vi "main.vi"() -> ()   [LabVIEW 2018]
uses:
  ControlEstados3.ctl
  <vilib>/MakerHub/LINX/Public/Peripherals/PWM/PWM Set Duty Cycle 1 Chan.vi
  <vilib>/MakerHub/LINX/Public/Utilities/Open Serial.vi
  <vilib>/MakerHub/LINX/Public/Peripherals/PWM/PWM Set Duty Cycle N Chans.vi
  <vilib>/MakerHub/LINX/LMH-LINX.lvlib
panel:
  out "Estado":T1
  in  "Máquina de estado":enum32{"LM35 RGB", "Hall sensor"}(tab)
  in  "Temperatura optima (led azul)":dbl=0.25 format="%#_13g"
  in  "Temperatura limite":dbl
  out "Color Box 2":u32(colorbox)
  out "Thermometer":dbl(slide) scale=0.0..100.0
  in  "lm35":bool
  in  "Parar lm35":bool
  out "hall indicator":bool
  in  "hall":bool
  in  "Parar hall":bool
  in  "Serial Port":refnum<visa-resource-name>="N/A"
  in  "stop":bool
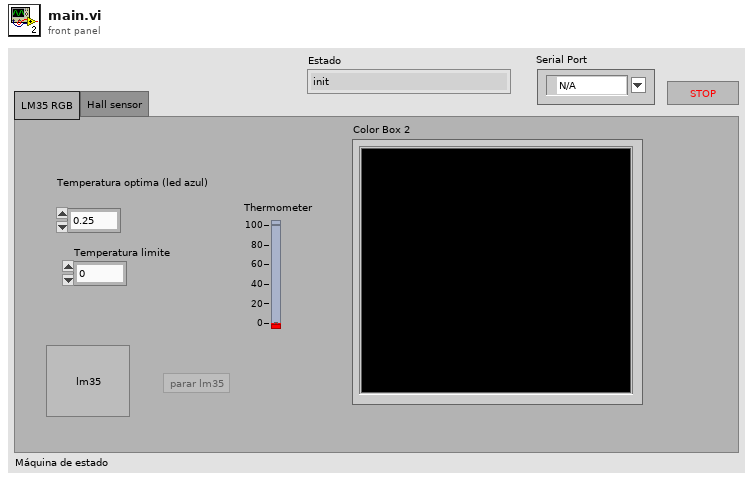
[diagram p1: front panel]
types:
  T1 = typedef "ControlEstados3.ctl" = enum16{"init", "wait for user event", "stop", "lm35", "hall"}
  T2 = enum8{"Enabled", "Disabled", "Disabled and Grayed Out"}
  T3 = typedef "LMH-LINX.lvlib/LINX Ref.ctl" = cluster{"IO":T4, "Interface":T5, "LINX Device Config":T6}
  T4 = typedef "LMH-LINX.lvlib/Platform.ctl" = enum16{"Remote", "Local"}
  T5 = typedef "LMH-LINX.lvlib/Interface.ctl" = enum16{"Serial", "TCP"}
  T6 = typedef "LMH-LINX.lvlib/Device.lvlib/LINX Device Config.ctl" = cluster{"Interface":T5, "COM Port":refnum<visa-resource-name>, "TCP Configuration":T7, "Device Family":u8, "Device ID":u8, "Device Name":string, "TCP Ref":refnum<k5>, "Channels":T8}
  T7 = typedef "LMH-LINX.lvlib/Device.lvlib/TCP Config.ctl" = cluster{"IP Address":string, "Port":u16}
  T8 = typedef "LMH-LINX.lvlib/Channels.ctl" = cluster{"DI":u8[], "DO":u8[], "AI":u8[], "AO":u8[], "PWM":u8[], "QE":u8[], "UART":u8[], "I2C 2":u8[], "SPI":u8[], "CAN":u8[], "Servo":u8[], "AI Ref (V)":dbl, "AI Resolution (Bits)":u8, "AO Ref (V)":dbl, "AO Resolution (Bits)":u8}
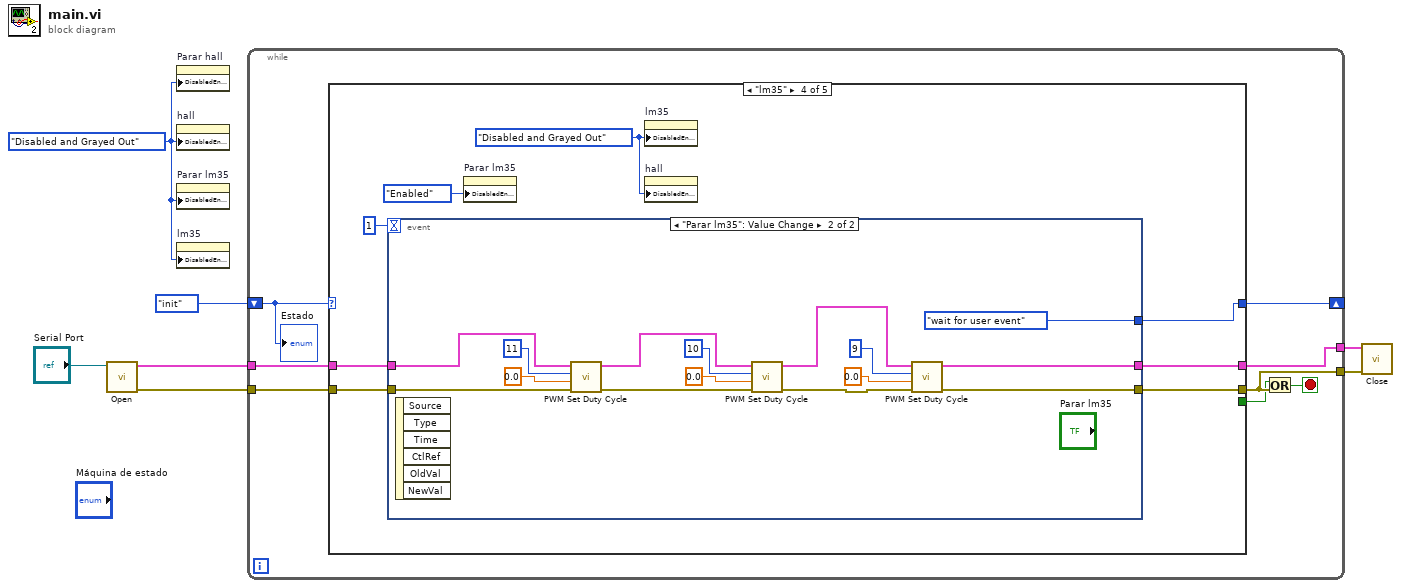
[diagram p0: block diagram]
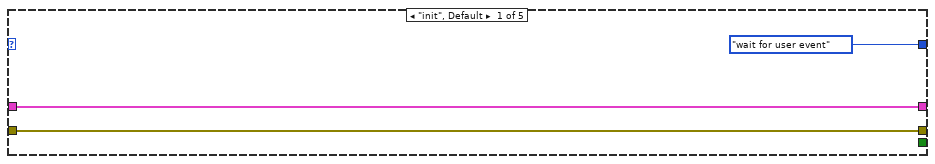
[diagram p2: hidden frame]
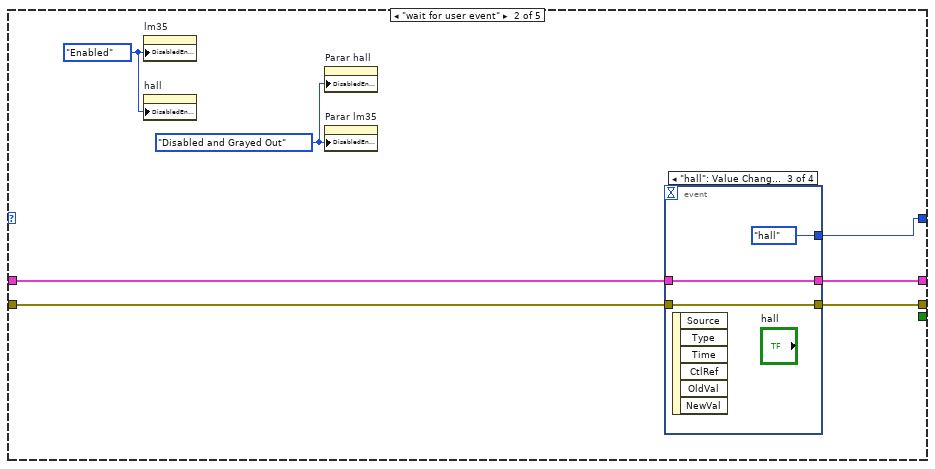
[diagram p3: hidden frame]
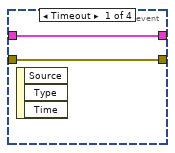
[diagram p4: hidden frame]
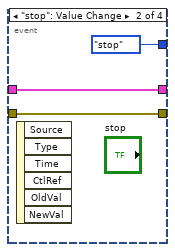
[diagram p5: hidden frame]
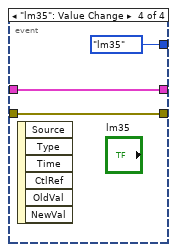
[diagram p6: hidden frame]
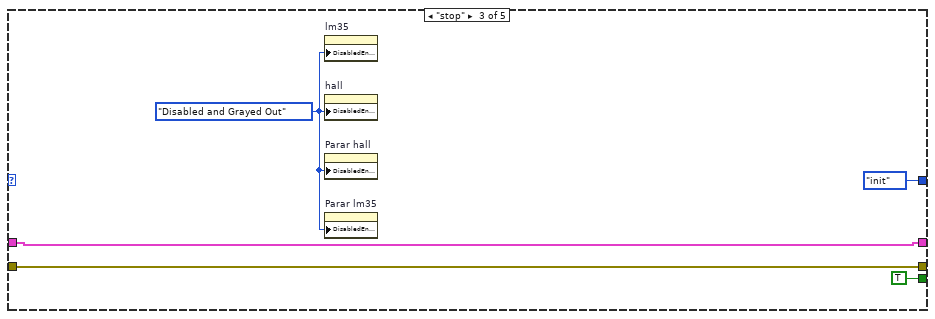
[diagram p7: hidden frame]
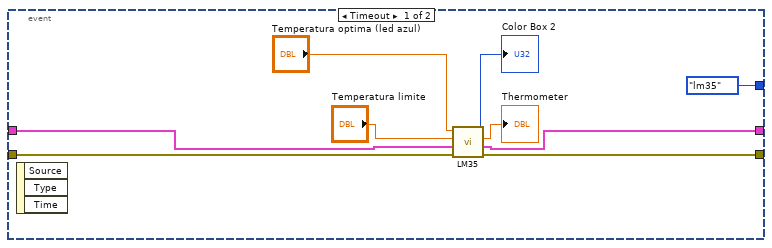
[diagram p8: hidden frame]
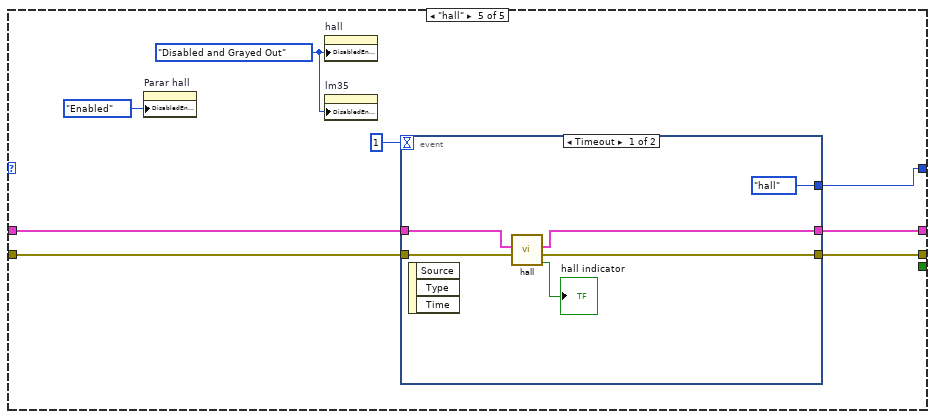
[diagram p9: hidden frame]
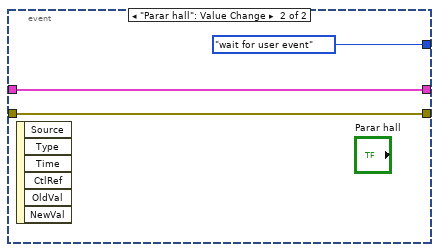
[diagram p10: hidden frame]
diagram:
  w1 = T2."Disabled and Grayed Out" ("Disabled")
  n1 = call-poly <vilib>:"Open.vi"("Serial Port"="Serial Port") -> ("Error Out"=w4:errorcluster, "LINX Resource"=w5:T3)  [unwired: 8 in, 1 out]
  n2 = property on="Parar hall" class="Bool"("DisabledEnum"=w1) -> ()  [unwired: 2 in, 2 out]
  n3 = property on="hall" class="Bool"("DisabledEnum"=w1) -> ()  [unwired: 2 in, 2 out]
  n4 = property on="Parar lm35" class="Bool"("DisabledEnum"=w1) -> ()  [unwired: 2 in, 2 out]
  n5 = property on="lm35" class="Bool"("DisabledEnum"=w1) -> ()  [unwired: 2 in, 2 out]
  n6 = while {
    shift-right: [w15] -> _
    shift-left: ControlEstados3."init" -> [w11]
    tunnel: w5 -> [w14]
    tunnel: w4 -> [w13]
    tunnel: [w12] -> w3
    tunnel: [w10] -> w2
    stop <- w8 stop-if-true
    n7 = case shown="\"lm35\"" w11 {
      tunnel: [ControlEstados3."wait for user event" w25 ControlEstados3."init" w49 w81] -> w15
      tunnel: [_ _ TRUE _ _] -> w9
      tunnel: w14 -> [w17 w23 w39 w46 w79]
      tunnel: w13 -> [w16 w21 w38 w44 w78]
      tunnel: [w17 w24 w39 w47 w77] -> w12
      tunnel: [w16 w22 w38 w45 w76] -> w10
      frame "init", Default {
      }
      frame "wait for user event" {
        w19 = T2."Disabled and Grayed Out" ("Disabled")
        w20 = T2."Enabled" ("Disabled")
        n8 = property on="lm35" class="Bool"("DisabledEnum"=w20) -> ()  [unwired: 2 in, 2 out]
        n9 = property on="hall" class="Bool"("DisabledEnum"=w20) -> ()  [unwired: 2 in, 2 out]
        n10 = property on="Parar hall" class="Bool"("DisabledEnum"=w19) -> ()  [unwired: 2 in, 2 out]
        n11 = property on="Parar lm35" class="Bool"("DisabledEnum"=w19) -> ()  [unwired: 2 in, 2 out]
        n12 = event shown="[2] \"hall\": Value Change" {
          selector: _ -> [_ _ _ _]
          dyn-events: _ -> [_ _ _ _]
          timeout: _ -> [_ _ _ _]
          tunnel: [_ ControlEstados3."stop" ControlEstados3."hall" ControlEstados3."lm35"] -> w25
          tunnel: [w27 w29 w32 w35] -> w24
          tunnel: w23 -> [w27 w29 w32 w35]
          tunnel: [w26 w28 w31 w34] -> w22
          tunnel: w21 -> [w26 w28 w31 w34]
          event Timeout {
            n13 = event-data() -> ()  [unwired: 1 in, 3 out]
          }
          event "stop": Value Change {
            n14 = event-data() -> ()  [unwired: 1 in, 6 out]
          }
          event "hall": Value Change {
            n15 = event-data() -> ()  [unwired: 1 in, 6 out]
          }
          event "lm35": Value Change {
            n16 = event-data() -> ()  [unwired: 1 in, 6 out]
          }
        }
      }
      frame "stop" {
        w37 = T2."Disabled and Grayed Out" ("Disabled")
        n17 = property on="lm35" class="Bool"("DisabledEnum"=w37) -> ()  [unwired: 2 in, 2 out]
        n18 = property on="hall" class="Bool"("DisabledEnum"=w37) -> ()  [unwired: 2 in, 2 out]
        n19 = property on="Parar hall" class="Bool"("DisabledEnum"=w37) -> ()  [unwired: 2 in, 2 out]
        n20 = property on="Parar lm35" class="Bool"("DisabledEnum"=w37) -> ()  [unwired: 2 in, 2 out]
      }
      frame "lm35" {
        w42 = T2."Disabled and Grayed Out" ("Disabled")
        n21 = event shown="[1] \"Parar lm35\": Value Change" {
          selector: _ -> [_ _]
          dyn-events: _ -> [_ _]
          timeout: 1 -> [_ _]
          tunnel: [ControlEstados3."lm35" ControlEstados3."wait for user event"] -> w49
          tunnel: [w51 w63] -> w47
          tunnel: w46 -> [w55 w66]
          tunnel: [w50 w59] -> w45
          tunnel: w44 -> [w54 w62]
          event Timeout {
            n22 = event-data() -> ()  [unwired: 1 in, 3 out]
            n23 = call "LM35.vi"("Error In"=w54, "LINX Resource"=w55, "temperatura limite"="Temperatura limite", "Temperatura optima (led azul)"="Temperatura optima (led azul)") -> ("Error Out"=w50:errorcluster, "LINX Resource 2"=w51:T3, "Thermometer"=→"Thermometer":dbl, "Color Box 2"=→"Color Box 2":u32)  [unwired: 4 in]
          }
          event "Parar lm35": Value Change {
            n24 = event-data() -> ()  [unwired: 1 in, 6 out]
            n25 = call-poly <vilib>:"PWM Set Duty Cycle.vi"("Error In"=w62, "Duty Cycle (0-1)"=0.0, "PWM Channel"=u8 11, "LINX Resource"=w66) -> ("Error Out"=w61:errorcluster, "LINX Resource"=w65:T3)  [unwired: 6 in]
            n26 = call-poly <vilib>:"PWM Set Duty Cycle.vi"("Error In"=w61, "Duty Cycle (0-1)"=0.0, "PWM Channel"=u8 10, "LINX Resource"=w65) -> ("Error Out"=w60:errorcluster, "LINX Resource"=w64:T3)  [unwired: 6 in]
            n27 = call-poly <vilib>:"PWM Set Duty Cycle.vi"("Error In"=w60, "Duty Cycle (0-1)"=0.0, "PWM Channel"=u8 9, "LINX Resource"=w64) -> ("Error Out"=w59:errorcluster, "LINX Resource"=w63:T3)  [unwired: 6 in]
          }
        }
        n28 = property on="Parar lm35" class="Bool"("DisabledEnum"=T2."Enabled" ("Disabled")) -> ()  [unwired: 2 in, 2 out]
        n29 = property on="lm35" class="Bool"("DisabledEnum"=w42) -> ()  [unwired: 2 in, 2 out]
        n30 = property on="hall" class="Bool"("DisabledEnum"=w42) -> ()  [unwired: 2 in, 2 out]
      }
      frame "hall" {
        w74 = T2."Disabled and Grayed Out" ("Disabled")
        n31 = property on="Parar hall" class="Bool"("DisabledEnum"=T2."Enabled" ("Disabled")) -> ()  [unwired: 2 in, 2 out]
        n32 = property on="hall" class="Bool"("DisabledEnum"=w74) -> ()  [unwired: 2 in, 2 out]
        n33 = property on="lm35" class="Bool"("DisabledEnum"=w74) -> ()  [unwired: 2 in, 2 out]
        n34 = event shown="[0] Timeout" {
          selector: _ -> [_ _]
          dyn-events: _ -> [_ _]
          timeout: 1 -> [_ _]
          tunnel: [ControlEstados3."hall" ControlEstados3."wait for user event"] -> w81
          tunnel: w79 -> [w85 w89]
          tunnel: w78 -> [w84 w88]
          tunnel: [w83 w89] -> w77
          tunnel: [w82 w88] -> w76
          event Timeout {
            n35 = event-data() -> ()  [unwired: 1 in, 3 out]
            n36 = call "hall.vi"("Error In"=w84, "LINX Resource"=w85) -> ("hall indicator"=→"hall indicator":bool, "Error Out"=w82:errorcluster, "LINX Resource 2"=w83:T3)  [unwired: 7 in]
          }
          event "Parar hall": Value Change {
            n37 = event-data() -> ()  [unwired: 1 in, 6 out]
          }
        }
      }
    }
    n38 = Or(x=w9, y=w10) -> (x .or. y?=w8:bool)
    "Estado" <- w11
  }
  n39 = call <vilib>:"Close.vi"("Error In"=w2, "LINX Resource"=w3) -> ()  [unwired: 9 in, 1 out]
